vi "api_Close.vi"(8 "error in (no error)":errorcluster, 11 "ConfigClass_DVR":refnum<data-value>) -> (0 "error out":errorcluster, 3 "ConfigClass_DVR_out":refnum<data-value>)   [LabVIEW 2019, in "ConfigClass.lvlib" / "ConfigClass.lvclass"]
uses:
  ConfigClass.lvclass
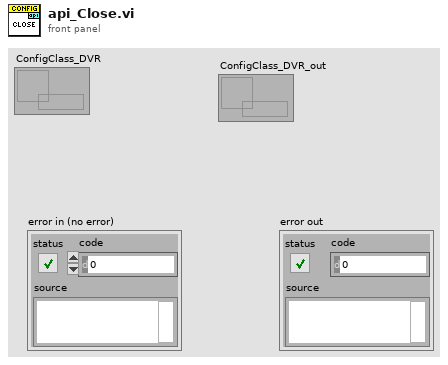
[diagram p1: front panel]
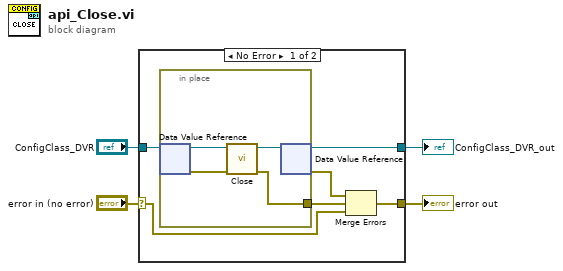
[diagram p0: block diagram]
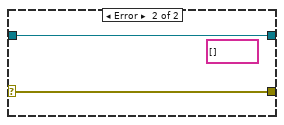
[diagram p2: hidden frame]
diagram:
  n1 = case shown="No Error" "error in (no error)" {
    selector: "error in (no error)" -> [w5 w16]
    tunnel: "ConfigClass_DVR" -> [w10 w15]
    tunnel: [w7 w16] -> w3
    tunnel: [w6 w15] -> w1
    frame No Error {
      n2 = in-place {
        in-place-border: [w11] -> w8
        n3 = in-place-dvr #1(w10) -> (w14:refnum<class "ConfigClass.lvclass">, w13:errorcluster)
        n4 = call-dynamic "Close.vi"("error in (no error)"=w13, "ConfigClass_IN"=w14) -> ("error out"=w11:errorcluster, "ConfigClass_OUT"=w12:refnum<class "ConfigClass.lvclass">)  [unwired: 8 in]
        n5 = in-place-dvr #1(w12) -> (w6:refnum<data-value>, w9:errorcluster)
      }
      n6 = Merge Errors(w9, w8, w5) -> (w7:errorcluster)
    }
    frame Error {
      (unwired) string[] [] ("params")
    }
  }
  "ConfigClass_DVR_out" <- w1
  "error out" <- w3
